vi "OLD Create.vi"(9 "Alias":string, 10 "Actor":refnum<class "Actor.lvclass">, 11 "jettl Queue Actor in":refnum<class "jettl Queue Actor.lvclass">) -> (3 "jettl Queue Actor out":refnum<class "jettl Queue Actor.lvclass">)   [LabVIEW 2021, in "jettl.lvlib" / "jettl Queue Actor.lvlib" / "jettl Queue Actor.lvclass"]
uses:
  jettl Queue Actor.lvclass
  C:/git/jettl/src/Actor/Actor/Actor.lvclass
  Actor/Actor/Actor.lvclass
  State/Nominal State/Nominal State.lvclass
  C:/git/jettl/src/jettl/jettl Queue Actor/State/State/State.lvclass
  jettl Queue Actor.lvclass/jettl Queue Actor.ctl
  Actor/Queue Actor/Loop.vi
  jettl.lvlib
  Actor/Queue Actor/Queue Actor.lvclass
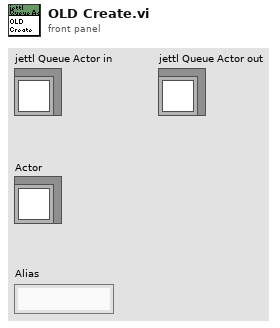
[diagram p1: front panel]
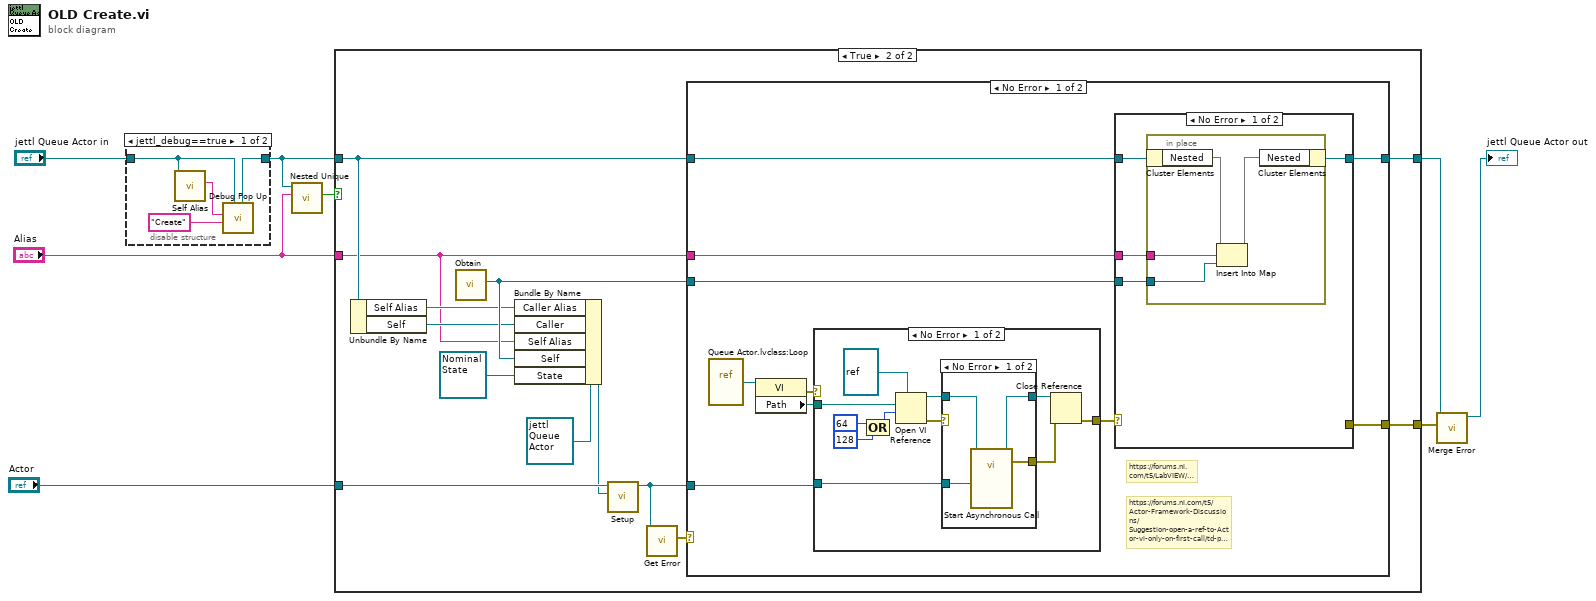
[diagram p0: block diagram]
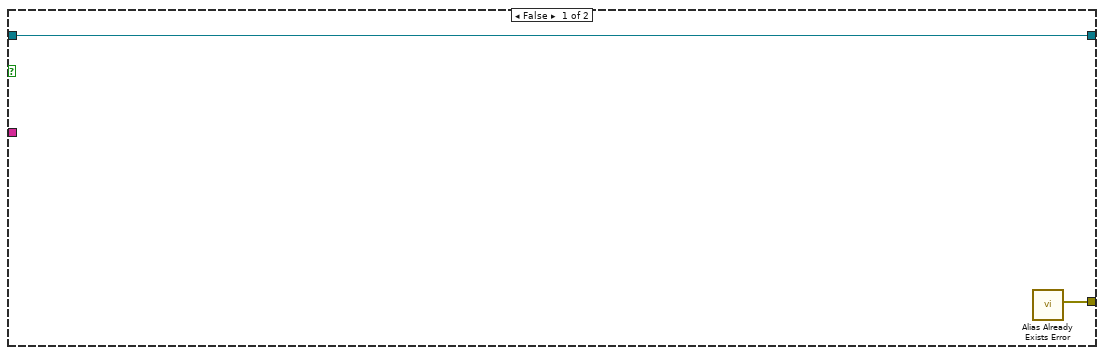
[diagram p3: hidden frame]
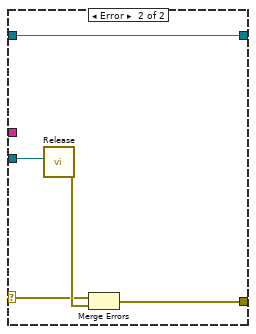
[diagram p6: hidden frame]
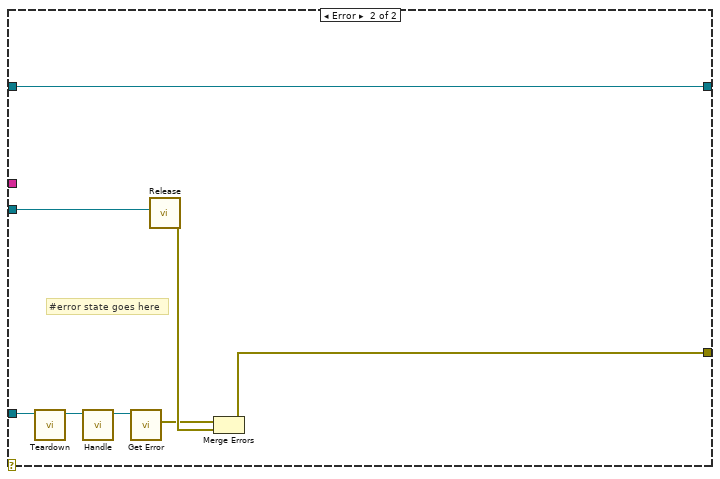
[diagram p7: hidden frame]
diagram:
  n1 = disable-structure shown="jettl_debug==true" {
    disable-tunnel: "jettl Queue Actor in" -> [w10 w13]
    disable-tunnel: [w12 w13] -> w3
    frame condition #0 (active) {
      n2 = call-dynamic "Self Alias.vi"("jettl Queue Actor in"=w10) -> ("Self Alias"=w9:string)  [unwired: 10 in]
      n3 = call "Debug Pop Up.vi"("Input"=w10, "Method"="Create", "Alias"=w9) -> ("Output"=w12:refnum<class "jettl Queue Actor.lvclass">)  [unwired: 8 in]
    }
    frame condition #1 {
    }
  }
  n4 = call-dynamic "Nested Unique.vi"("Nested Alias"="Alias", "jettl Queue Actor in"=w3) -> ("Nested Alias Unique?"=w7:bool)  [unwired: 9 in]
  n5 = case shown="True" w7 {
    tunnel: "Actor" -> [_ w28]
    tunnel: [w15 w24] -> w5
    tunnel: w3 -> [w15 w26]
    tunnel: "Alias" -> [_ w16]
    tunnel: [w14 w25] -> w6
    frame False {
      n6 = call "Alias Already Exists Error.vi"() -> ("Error"=w14:errorcluster)  [unwired: 11 in]
    }
    frame True {
      n7 = Unbundle By Name(w26) -> ("Self Alias"=w20:string, "Self"=w21:refnum<data-value>)
      n8 = call "Obtain.vi"() -> ("Queue"=w27:refnum<data-value>)  [unwired: 10 in, 1 out]
      n9 = Bundle By Name(cluster=refnum<class "jettl Queue Actor.lvclass"> refnum ("Self Actor in"), "Caller Alias"=w20, "Caller"=w21, "Self Alias"=w16, "Self"=w27, "State"=refnum<class "Nominal State.lvclass"> refnum ("LVCAM.lvlib:Msging Self Actor State.lvclass")) -> (w17:refnum<class "jettl Queue Actor.lvclass">)
      n10 = call-dynamic "Setup.vi"("Actor"=w17, "Actor in"=w28) -> ("Actor out"=w22:refnum<class "Actor.lvclass">)  [unwired: 9 in]
      n11 = call-dynamic "Get Error.vi"("Actor in"=w22) -> ("Error"=w23:errorcluster)  [unwired: 10 in]
      n12 = case shown="No Error" w23 {
        tunnel: [w38 w76] -> w24
        tunnel: w22 -> [w37 w74]
        tunnel: [w36 w75] -> w25
        tunnel: w26 -> [w34 w76]
        tunnel: w27 -> [w33 w77]
        tunnel: w16 -> [w29 _]
        frame No Error {
          # "https://forums.ni.com/t5/LabVIEW/Static-VI-Reference/m-p/3334014#M978333"
          # "https://forums.ni.com/t5/Actor-Framework-Discussions/Suggestion-open-a-ref-to-Actor-vi-only-on-first-call/td-p/3451643/page/4"
          n13 = vi-ref "Queue Actor.lvclass:Loop.vi"() -> (w31:refnum<vi>)
          n14 = property class="VI"(reference=w31) -> (error out=w32:errorcluster, "Path"=w30:path)  [unwired: 1 in, 1 out]
          n15 = case shown="No Error" w32 {
            selector: w32 -> [_ w56]
            tunnel: [w47 w56] -> w35
            tunnel: w30 -> [w43 _]
            tunnel: w37 -> [w39 _]
            frame No Error {
              n16 = Compound Arithmetic op=OR(64 ("options: Multiple Clones,\n  Fire & Forget"), 128 ("options: Multiple Clones,\n  Fire & Forget")) -> (w45:i32)
              n17 = Open VI Reference(type specifier VI Refnum (for type only)=refnum<vi> refnum, vi path=w43, options=w45) -> (vi reference=w41:refnum<vi>, error out=w42:errorcluster)  [unwired: 3 in]
              n18 = case shown="No Error" w42 {
                selector: w42 -> [_ w55]
                tunnel: [w53 w54] -> w49
                tunnel: [w52 w55] -> w48
                tunnel: w41 -> [w51 w54]
                tunnel: w39 -> [w50 _]
                frame No Error {
                  n19 = call-by-ref "Start Asynchronous Call"(reference=w51, "Actor"=w50) -> (reference out=w53:refnum<vi>, error out=w52:errorcluster)  [unwired: 12 in]
                }
                frame Error {
                }
              }
              n20 = Close Reference(reference=w49, error in (no error)=w48) -> (error out=w47:errorcluster)
            }
            frame Error {
            }
          }
          n21 = case shown="No Error" w35 {
            selector: w35 -> [_ w65]
            tunnel: w34 -> [w60 w69]
            tunnel: [w59 w69] -> w38
            tunnel: w33 -> [w58 w68]
            tunnel: [_ w67] -> w36
            tunnel: w29 -> [w57 _]
            frame No Error {
              n22 = in-place {
                in-place-border: w58 -> [w62]
                in-place-border: w57 -> [w61]
                n23 = in-place-cluster #1(w60) -> ("Nested"=w64:map{string, refnum<data-value>})
                n24 = Insert Into Map(map in=w64, key=w61, value=w62) -> (map out=w63:map{string, refnum<data-value>})  [unwired: 2 out]
                n25 = in-place-cluster #1("Nested"=w63) -> (w59:refnum<class "jettl Queue Actor.lvclass">)
              }
            }
            frame Error {
              n26 = call "Release.vi"("Queue"=w68) -> ("error out"=w66:errorcluster)  [unwired: 10 in]
              n27 = Merge Errors(w65, w66) -> (w67:errorcluster)
            }
          }
        }
        frame Error {
          # "#error state goes here"
          n28 = call-dynamic "Teardown.vi"("Teardown in"=w74) -> ("Teardown out"=w73:refnum<class "Actor.lvclass">)  [unwired: 10 in]
          n29 = call-dynamic "Handle.vi"("Actor in"=w73) -> ("Actor out"=w72:refnum<class "Actor.lvclass">)  [unwired: 9 in, 1 out]
          n30 = call-dynamic "Get Error.vi"("Actor in"=w72) -> ("Error"=w70:errorcluster)  [unwired: 10 in]
          n31 = call "Release.vi"("Queue"=w77) -> ("error out"=w71:errorcluster)  [unwired: 10 in]
          n32 = Merge Errors(w70, w71) -> (w75:errorcluster)
        }
      }
    }
  }
  n33 = call-dynamic "Merge Error.vi"("Error"=w6, "jettl Queue Actor in"=w5) -> ("jettl Queue Actor out"=→"jettl Queue Actor out":refnum<class "jettl Queue Actor.lvclass">)  [unwired: 9 in]
